vi "PAS_read_voltage.vi"(8 "error in (no error)":errorcluster, 10 "Hi-res Mode":bool, 11 "VISA Refnum in":refnum<visa-resource-name>) -> (0 "error out":errorcluster, 1 "voltage (double)":dbl, 2 "voltage (String)":string, 3 "VISA Refnum out":refnum<visa-resource-name>)   [LabVIEW 2020]
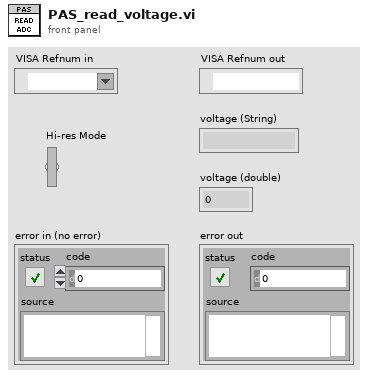
[diagram p1: front panel]
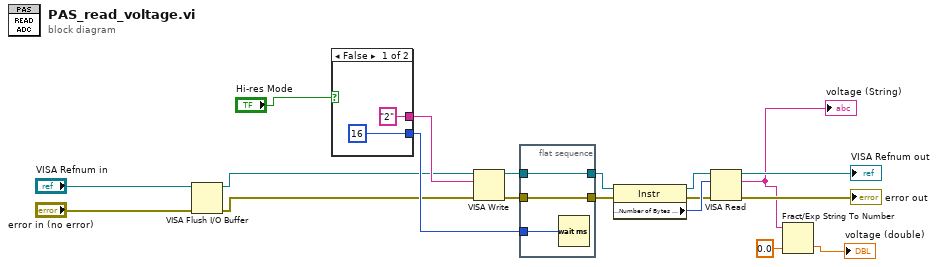
[diagram p0: block diagram]
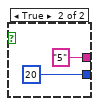
[diagram p2: hidden frame]
diagram:
  n1 = VISA Flush I/O Buffer(VISA resource name="VISA Refnum in", error in (no error)="error in (no error)") -> (VISA resource name out=w2:refnum<visa-resource-name>, error out=w1:errorcluster)  [unwired: 1 in]
  n2 = case shown="False" "Hi-res Mode" {
    tunnel: ["2" ("write buffer") "5" ("write buffer")] -> w10
    tunnel: [u32 16 ("milliseconds to wait") u32 20 ("milliseconds to wait")] -> w5
    frame False {
    }
    frame True {
    }
  }
  n3 = VISA Write(VISA resource name=w2, write buffer=w10, error in (no error)=w1) -> (VISA resource name out=w11:refnum<visa-resource-name>, error out=w12:errorcluster)  [unwired: 1 out]
  n4 = flat-sequence {
    tunnel: w11 -> [w26]
    tunnel: [w26] -> w15
    tunnel: w12 -> [w25]
    tunnel: [w25] -> w13
    tunnel: w5 -> [w24]
    frame #0 {
      n5 = Wait (ms)(milliseconds to wait=w24) -> ()  [unwired: 1 out]
    }
  }
  n6 = property class="Instr"(reference=w15, error in=w13) -> (reference out=w16:refnum<visa-resource-name>, error out=w14:errorcluster, "Serial Settings:Number of Bytes at Serial Port"=w17:u32)
  n7 = VISA Read(VISA resource name=w16, byte count=w17, error in (no error)=w14) -> (VISA resource name out=→"VISA Refnum out":refnum<visa-resource-name>, read buffer=w9:string, error out=→"error out":errorcluster)  [unwired: 1 out]
  "voltage (String)" <- w9
  n8 = Fract/Exp String To Number(string=w9, default (0 dbl)=0.0 ("default (0 I32)")) -> (number=→"voltage (double)":dbl)  [unwired: 2 in, 1 out]
